vi "CollectData.vi"(8 "error in (no error)":errorcluster, 11 "SRS_SG380 in":refnum<class "SRS_SG380.lvclass">) -> (0 "error out":errorcluster, 3 "SRS_SG380 out":refnum<class "SRS_SG380.lvclass">)   [LabVIEW 2013, in "SRS_SG380.lvclass"]
uses:
  SRS_SG380.lvclass
  Device/Device.lvclass
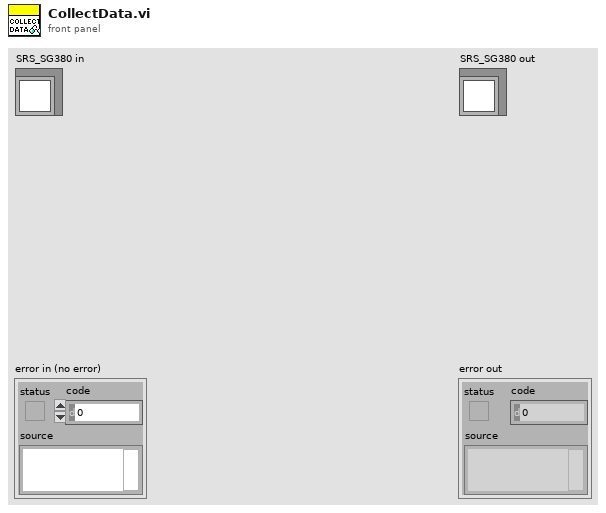
[diagram p1: front panel]
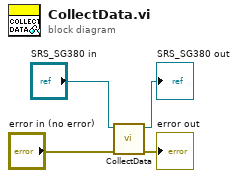
[diagram p0: block diagram]
diagram:
  n1 = call-parent "CollectData.vi"("error in (no error)"="error in (no error)", "Device in"="SRS_SG380 in") -> ("error out"=→"error out":errorcluster, "Device out"=→"SRS_SG380 out":refnum<class "SRS_SG380.lvclass">)  [unwired: 8 in]
